vi "Parse Property Bundle.vi"(10 "Name":string, 11 "Property Bundle":cluster{"Name":string, "Value":variant}[](array[cluster])) -> (2 "Found?":bool, 3 "Value":variant)   [LabVIEW 2021]
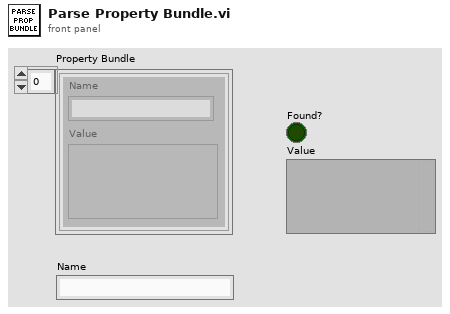
[diagram p1: front panel]
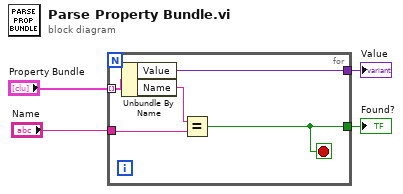
[diagram p0: block diagram]
diagram:
  n1 = for {
    tunnel: "Property Bundle" -> [w9] mode=indexing
    tunnel: "Name" -> [w7]
    tunnel: [w6] -> w1
    tunnel: [w5] -> w2
    stop <- w5 stop-if-true
    n2 = Unbundle By Name(w9) -> ("Value"=w6:variant, "Name"=w8:string)
    n3 = Equal?(x=w8, y=w7) -> (x = y?=w5:bool)
  }
  "Found?" <- w2
  "Value" <- w1
